vi "getICCamAcq.vi"(8 "error in (no error)":errorcluster, 11 "ICCameraController in":refnum<class "ICCameraController.lvclass">) -> (0 "error out":errorcluster, 2 "ICCameraAcquisitor":refnum<class "ICCameraAcquisitor.lvclass">, 3 "ICCameraController out":refnum<class "ICCameraController.lvclass">)   [LabVIEW 2009, in "Hardware.lvlib" / "Channels.lvlib" / "ICCameraController.lvclass"]
uses:
  ICCameraController.lvclass
  ICCameraAcquisitor/ICCameraAcquisitor.lvclass
  ICCameraController.lvclass/ICCameraController.ctl
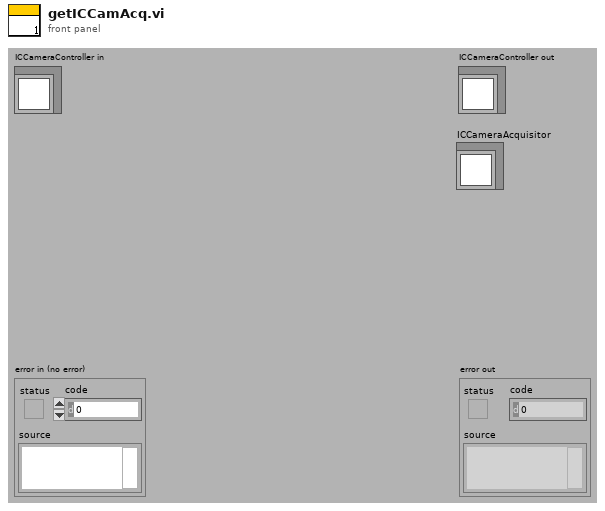
[diagram p1: front panel]
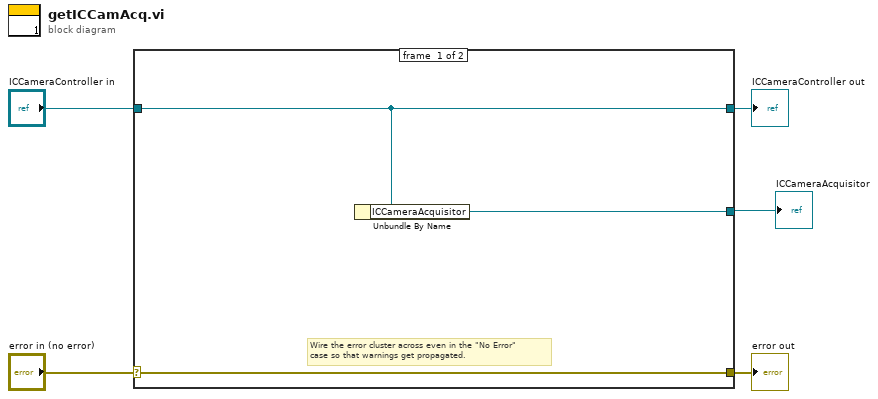
[diagram p0: block diagram]
diagram:
  n1 = case shown="No Error" "error in (no error)" {
    selector: "error in (no error)" -> [w8 w10]
    tunnel: [w8 w10] -> w4
    tunnel: [w7 w9] -> w2
    tunnel: "ICCameraController in" -> [w7 w9]
    tunnel: [w6 _] -> w1
    frame #0 {
      # "Wire the error cluster across even in the \"No Error\"\ncase so that warnings get propagated."
      n2 = Unbundle By Name(w7) -> ("ICCameraAcquisitor"=w6:refnum<class "ICCameraAcquisitor.lvclass">)
    }
    frame #1 {
    }
  }
  "error out" <- w4
  "ICCameraController out" <- w2
  "ICCameraAcquisitor" <- w1
